vi "Cervena-Narozeninova.vi"(11 "NXT/EV3":T1) -> (3 "NXT/EV3 2":T1)   [LabVIEW 2016]
uses:
  <vilib>/NXT/Subs/LVHSConnector.ctl
  <vilib>/NXT/LegoClasses/BrickReference/BrickReference.lvclass
  <vilib>/NXT/Dual Mode Library/Sound/PlayG.vi
  <vilib>/NXT/Dual Mode Library/Sound/PlayF.vi
  <vilib>/NXT/Dual Mode Library/Sound/PlayE.vi
  <vilib>/NXT/Dual Mode Library/Waits/Wait_Num.vi
  <vilib>/NXT/Dual Mode Library/Sound/PlayA.vi
  <vilib>/NXT/Dual Mode Library/Sound/PlayB.vi
  <vilib>/NXT/Dual Mode Library/Sound/PlayC.vi
  <vilib>/NXT/Dual Mode Library/Sound/PlayD.vi
  <vilib>/NXT/Dual Mode Library/Display/drawText_Center.vi
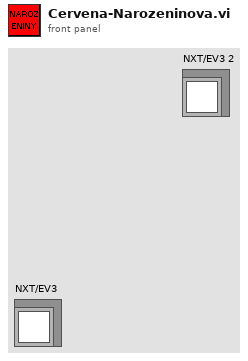
[diagram p1: front panel]
types:
  T1 = typedef "LVHSConnector.ctl" = refnum<class "BrickReference.lvclass">
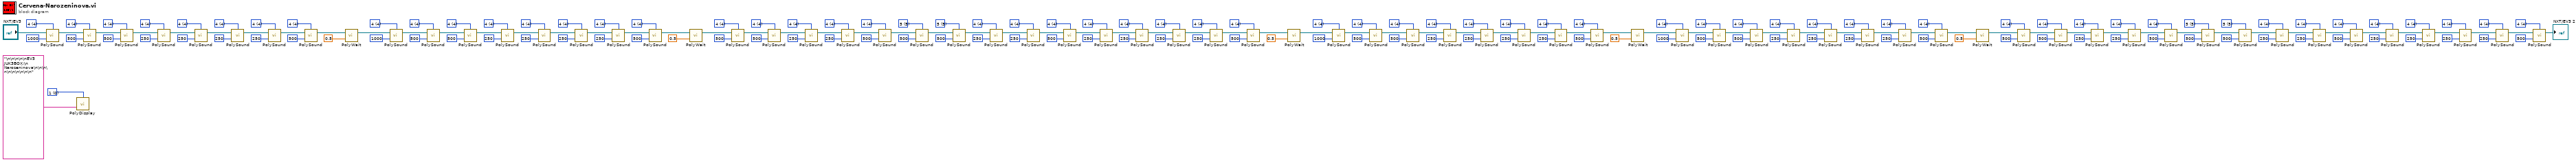
[diagram p0: block diagram]
diagram:
  w1 = i16 0 items=["1", "2", "3", "4", "5", "6", "7", "8", "9", "10", "11", "12"] ("Line")
  w11 = u16 4 items=["3"=3, "4"=4, "5"=5, "6"=6, "7"=7] ("Octave")
  w17 = u16 4 items=["3"=3, "4"=4, "5"=5, "6"=6, "7"=7] ("Octave")
  w16 = u16 4 items=["3"=3, "4"=4, "5"=5, "6"=6, "7"=7] ("Octave")
  w18 = u16 4 items=["3"=3, "4"=4, "5"=5, "6"=6, "7"=7] ("Octave")
  w19 = u16 4 items=["3"=3, "4"=4, "5"=5, "6"=6, "7"=7] ("Octave")
  w27 = u16 4 items=["3"=3, "4"=4, "5"=5, "6"=6, "7"=7] ("Octave")
  w28 = u16 4 items=["3"=3, "4"=4, "5"=5, "6"=6, "7"=7] ("Octave")
  w31 = u16 4 items=["3"=3, "4"=4, "5"=5, "6"=6, "7"=7] ("Octave")
  w33 = u16 5 items=["3"=3, "4"=4, "5"=5, "6"=6, "7"=7] ("Octave")
  w45 = u16 5 items=["3"=3, "4"=4, "5"=5, "6"=6, "7"=7] ("Octave")
  w46 = u16 4 items=["3"=3, "4"=4, "5"=5, "6"=6, "7"=7] ("Octave")
  w49 = u16 4 items=["3"=3, "4"=4, "5"=5, "6"=6, "7"=7] ("Octave")
  w50 = u16 4 items=["3"=3, "4"=4, "5"=5, "6"=6, "7"=7] ("Octave")
  w52 = u16 4 items=["3"=3, "4"=4, "5"=5, "6"=6, "7"=7] ("Octave")
  w55 = u16 4 items=["3"=3, "4"=4, "5"=5, "6"=6, "7"=7] ("Octave")
  w79 = u16 4 items=["3"=3, "4"=4, "5"=5, "6"=6, "7"=7] ("Octave")
  w73 = u16 4 items=["3"=3, "4"=4, "5"=5, "6"=6, "7"=7] ("Octave")
  w72 = u16 4 items=["3"=3, "4"=4, "5"=5, "6"=6, "7"=7] ("Octave")
  w68 = u16 4 items=["3"=3, "4"=4, "5"=5, "6"=6, "7"=7] ("Octave")
  w69 = u16 4 items=["3"=3, "4"=4, "5"=5, "6"=6, "7"=7] ("Octave")
  w62 = u16 4 items=["3"=3, "4"=4, "5"=5, "6"=6, "7"=7] ("Octave")
  w61 = u16 4 items=["3"=3, "4"=4, "5"=5, "6"=6, "7"=7] ("Octave")
  w58 = u16 4 items=["3"=3, "4"=4, "5"=5, "6"=6, "7"=7] ("Octave")
  w82 = u16 4 items=["3"=3, "4"=4, "5"=5, "6"=6, "7"=7] ("Octave")
  w88 = u16 4 items=["3"=3, "4"=4, "5"=5, "6"=6, "7"=7] ("Octave")
  w89 = u16 4 items=["3"=3, "4"=4, "5"=5, "6"=6, "7"=7] ("Octave")
  w93 = u16 4 items=["3"=3, "4"=4, "5"=5, "6"=6, "7"=7] ("Octave")
  w92 = u16 4 items=["3"=3, "4"=4, "5"=5, "6"=6, "7"=7] ("Octave")
  w99 = u16 4 items=["3"=3, "4"=4, "5"=5, "6"=6, "7"=7] ("Octave")
  w100 = u16 4 items=["3"=3, "4"=4, "5"=5, "6"=6, "7"=7] ("Octave")
  w103 = u16 4 items=["3"=3, "4"=4, "5"=5, "6"=6, "7"=7] ("Octave")
  w107 = u16 4 items=["3"=3, "4"=4, "5"=5, "6"=6, "7"=7] ("Octave")
  w113 = u16 4 items=["3"=3, "4"=4, "5"=5, "6"=6, "7"=7] ("Octave")
  w112 = u16 4 items=["3"=3, "4"=4, "5"=5, "6"=6, "7"=7] ("Octave")
  w114 = u16 4 items=["3"=3, "4"=4, "5"=5, "6"=6, "7"=7] ("Octave")
  w115 = u16 4 items=["3"=3, "4"=4, "5"=5, "6"=6, "7"=7] ("Octave")
  w123 = u16 4 items=["3"=3, "4"=4, "5"=5, "6"=6, "7"=7] ("Octave")
  w124 = u16 4 items=["3"=3, "4"=4, "5"=5, "6"=6, "7"=7] ("Octave")
  w127 = u16 4 items=["3"=3, "4"=4, "5"=5, "6"=6, "7"=7] ("Octave")
  w129 = u16 5 items=["3"=3, "4"=4, "5"=5, "6"=6, "7"=7] ("Octave")
  w141 = u16 5 items=["3"=3, "4"=4, "5"=5, "6"=6, "7"=7] ("Octave")
  w142 = u16 4 items=["3"=3, "4"=4, "5"=5, "6"=6, "7"=7] ("Octave")
  w145 = u16 4 items=["3"=3, "4"=4, "5"=5, "6"=6, "7"=7] ("Octave")
  w146 = u16 4 items=["3"=3, "4"=4, "5"=5, "6"=6, "7"=7] ("Octave")
  w148 = u16 4 items=["3"=3, "4"=4, "5"=5, "6"=6, "7"=7] ("Octave")
  w151 = u16 4 items=["3"=3, "4"=4, "5"=5, "6"=6, "7"=7] ("Octave")
  w175 = u16 4 items=["3"=3, "4"=4, "5"=5, "6"=6, "7"=7] ("Octave")
  w169 = u16 4 items=["3"=3, "4"=4, "5"=5, "6"=6, "7"=7] ("Octave")
  w168 = u16 4 items=["3"=3, "4"=4, "5"=5, "6"=6, "7"=7] ("Octave")
  w164 = u16 4 items=["3"=3, "4"=4, "5"=5, "6"=6, "7"=7] ("Octave")
  w165 = u16 4 items=["3"=3, "4"=4, "5"=5, "6"=6, "7"=7] ("Octave")
  w158 = u16 4 items=["3"=3, "4"=4, "5"=5, "6"=6, "7"=7] ("Octave")
  w157 = u16 4 items=["3"=3, "4"=4, "5"=5, "6"=6, "7"=7] ("Octave")
  w154 = u16 4 items=["3"=3, "4"=4, "5"=5, "6"=6, "7"=7] ("Octave")
  w178 = u16 4 items=["3"=3, "4"=4, "5"=5, "6"=6, "7"=7] ("Octave")
  w184 = u16 4 items=["3"=3, "4"=4, "5"=5, "6"=6, "7"=7] ("Octave")
  w185 = u16 4 items=["3"=3, "4"=4, "5"=5, "6"=6, "7"=7] ("Octave")
  w189 = u16 4 items=["3"=3, "4"=4, "5"=5, "6"=6, "7"=7] ("Octave")
  w188 = u16 4 items=["3"=3, "4"=4, "5"=5, "6"=6, "7"=7] ("Octave")
  w195 = u16 4 items=["3"=3, "4"=4, "5"=5, "6"=6, "7"=7] ("Octave")
  w196 = u16 4 items=["3"=3, "4"=4, "5"=5, "6"=6, "7"=7] ("Octave")
  w199 = u16 4 items=["3"=3, "4"=4, "5"=5, "6"=6, "7"=7] ("Octave")
  n1 = call-poly <vilib>:"PolySound.vi"("Duration (500 ms)"=u16 1000, "NXT/EV3"="NXT/EV3", "Octave"=w199) -> ("NXT/EV3"=w193:T1)  [unwired: 1 in]
  n2 = call-poly <vilib>:"PolyDisplay.vi"("Text"="\n\n\n\n\nEV3 JUK3BOX:\n Narozeninova\n\n\n\n\n\n\n\n\n\n", "Line"=w1) -> ()  [unwired: 2 in, 1 out]
  n3 = call-poly <vilib>:"PolySound.vi"("Duration (500 ms)"=u16 500, "NXT/EV3"=w193, "Octave"=w196) -> ("NXT/EV3"=w192:T1)  [unwired: 1 in]
  n4 = call-poly <vilib>:"PolySound.vi"("Duration (500 ms)"=u16 500, "NXT/EV3"=w192, "Octave"=w195) -> ("NXT/EV3"=w180:T1)  [unwired: 1 in]
  n5 = call-poly <vilib>:"PolySound.vi"("Duration (500 ms)"=u16 250, "NXT/EV3"=w180, "Octave"=w188) -> ("NXT/EV3"=w191:T1)  [unwired: 1 in]
  n6 = call-poly <vilib>:"PolySound.vi"("Duration (500 ms)"=u16 250, "NXT/EV3"=w191, "Octave"=w189) -> ("NXT/EV3"=w181:T1)  [unwired: 1 in]
  n7 = call-poly <vilib>:"PolySound.vi"("Duration (500 ms)"=u16 250, "NXT/EV3"=w181, "Octave"=w185) -> ("NXT/EV3"=w182:T1)  [unwired: 1 in]
  n8 = call-poly <vilib>:"PolySound.vi"("Duration (500 ms)"=u16 250, "NXT/EV3"=w182, "Octave"=w184) -> ("NXT/EV3"=w177:T1)  [unwired: 1 in]
  n9 = call-poly <vilib>:"PolySound.vi"("Duration (500 ms)"=u16 500, "NXT/EV3"=w177, "Octave"=w178) -> ("NXT/EV3"=w131:T1)  [unwired: 1 in]
  n10 = call-poly <vilib>:"PolyWait.vi"("Time (1 sec)"=sgl 0.5, "NXT/EV3"=w131) -> ("NXT/EV3"=w153:T1)  [unwired: 2 in]
  n11 = call-poly <vilib>:"PolySound.vi"("Duration (500 ms)"=u16 1000, "NXT/EV3"=w153, "Octave"=w154) -> ("NXT/EV3"=w160:T1)  [unwired: 1 in]
  n12 = call-poly <vilib>:"PolySound.vi"("Duration (500 ms)"=u16 500, "NXT/EV3"=w160, "Octave"=w157) -> ("NXT/EV3"=w161:T1)  [unwired: 1 in]
  n13 = call-poly <vilib>:"PolySound.vi"("Duration (500 ms)"=u16 500, "NXT/EV3"=w161, "Octave"=w158) -> ("NXT/EV3"=w173:T1)  [unwired: 1 in]
  n14 = call-poly <vilib>:"PolySound.vi"("Duration (500 ms)"=u16 250, "NXT/EV3"=w173, "Octave"=w165) -> ("NXT/EV3"=w162:T1)  [unwired: 1 in]
  n15 = call-poly <vilib>:"PolySound.vi"("Duration (500 ms)"=u16 250, "NXT/EV3"=w162, "Octave"=w164) -> ("NXT/EV3"=w172:T1)  [unwired: 1 in]
  n16 = call-poly <vilib>:"PolySound.vi"("Duration (500 ms)"=u16 250, "NXT/EV3"=w172, "Octave"=w168) -> ("NXT/EV3"=w171:T1)  [unwired: 1 in]
  n17 = call-poly <vilib>:"PolySound.vi"("Duration (500 ms)"=u16 250, "NXT/EV3"=w171, "Octave"=w169) -> ("NXT/EV3"=w176:T1)  [unwired: 1 in]
  n18 = call-poly <vilib>:"PolySound.vi"("Duration (500 ms)"=u16 500, "NXT/EV3"=w176, "Octave"=w175) -> ("NXT/EV3"=w133:T1)  [unwired: 1 in]
  n19 = call-poly <vilib>:"PolyWait.vi"("Time (1 sec)"=sgl 0.5, "NXT/EV3"=w133) -> ("NXT/EV3"=w132:T1)  [unwired: 2 in]
  n20 = call-poly <vilib>:"PolySound.vi"("Duration (500 ms)"=u16 500, "NXT/EV3"=w132, "Octave"=w151) -> ("NXT/EV3"=w139:T1)  [unwired: 1 in]
  n21 = call-poly <vilib>:"PolySound.vi"("Duration (500 ms)"=u16 500, "NXT/EV3"=w139, "Octave"=w148) -> ("NXT/EV3"=w138:T1)  [unwired: 1 in]
  n22 = call-poly <vilib>:"PolySound.vi"("Duration (500 ms)"=u16 250, "NXT/EV3"=w138, "Octave"=w146) -> ("NXT/EV3"=w137:T1)  [unwired: 1 in]
  n23 = call-poly <vilib>:"PolySound.vi"("Duration (500 ms)"=u16 250, "NXT/EV3"=w137, "Octave"=w145) -> ("NXT/EV3"=w136:T1)  [unwired: 1 in]
  n24 = call-poly <vilib>:"PolySound.vi"("Duration (500 ms)"=u16 500, "NXT/EV3"=w136, "Octave"=w142) -> ("NXT/EV3"=w135:T1)  [unwired: 1 in]
  n25 = call-poly <vilib>:"PolySound.vi"("Duration (500 ms)"=u16 500, "NXT/EV3"=w135, "Octave"=w141) -> ("NXT/EV3"=w128:T1)  [unwired: 1 in]
  n26 = call-poly <vilib>:"PolySound.vi"("Duration (500 ms)"=u16 500, "NXT/EV3"=w128, "Octave"=w129) -> ("NXT/EV3"=w121:T1)  [unwired: 1 in]
  n27 = call-poly <vilib>:"PolySound.vi"("Duration (500 ms)"=u16 250, "NXT/EV3"=w121, "Octave"=w127) -> ("NXT/EV3"=w120:T1)  [unwired: 1 in]
  n28 = call-poly <vilib>:"PolySound.vi"("Duration (500 ms)"=u16 250, "NXT/EV3"=w120, "Octave"=w124) -> ("NXT/EV3"=w119:T1)  [unwired: 1 in]
  n29 = call-poly <vilib>:"PolySound.vi"("Duration (500 ms)"=u16 500, "NXT/EV3"=w119, "Octave"=w123) -> ("NXT/EV3"=w106:T1)  [unwired: 1 in]
  n30 = call-poly <vilib>:"PolySound.vi"("Duration (500 ms)"=u16 250, "NXT/EV3"=w106, "Octave"=w115) -> ("NXT/EV3"=w118:T1)  [unwired: 1 in]
  n31 = call-poly <vilib>:"PolySound.vi"("Duration (500 ms)"=u16 250, "NXT/EV3"=w118, "Octave"=w114) -> ("NXT/EV3"=w105:T1)  [unwired: 1 in]
  n32 = call-poly <vilib>:"PolySound.vi"("Duration (500 ms)"=u16 250, "NXT/EV3"=w105, "Octave"=w112) -> ("NXT/EV3"=w109:T1)  [unwired: 1 in]
  n33 = call-poly <vilib>:"PolySound.vi"("Duration (500 ms)"=u16 250, "NXT/EV3"=w109, "Octave"=w113) -> ("NXT/EV3"=w104:T1)  [unwired: 1 in]
  n34 = call-poly <vilib>:"PolySound.vi"("Duration (500 ms)"=u16 500, "NXT/EV3"=w104, "Octave"=w107) -> ("NXT/EV3"=w7:T1)  [unwired: 1 in]
  n35 = call-poly <vilib>:"PolyWait.vi"("Time (1 sec)"=sgl 0.5, "NXT/EV3"=w7) -> ("NXT/EV3"=w6:T1)  [unwired: 2 in]
  n36 = call-poly <vilib>:"PolySound.vi"("Duration (500 ms)"=u16 1000, "NXT/EV3"=w6, "Octave"=w103) -> ("NXT/EV3"=w97:T1)  [unwired: 1 in]
  n37 = call-poly <vilib>:"PolySound.vi"("Duration (500 ms)"=u16 500, "NXT/EV3"=w97, "Octave"=w100) -> ("NXT/EV3"=w96:T1)  [unwired: 1 in]
  n38 = call-poly <vilib>:"PolySound.vi"("Duration (500 ms)"=u16 500, "NXT/EV3"=w96, "Octave"=w99) -> ("NXT/EV3"=w84:T1)  [unwired: 1 in]
  n39 = call-poly <vilib>:"PolySound.vi"("Duration (500 ms)"=u16 250, "NXT/EV3"=w84, "Octave"=w92) -> ("NXT/EV3"=w95:T1)  [unwired: 1 in]
  n40 = call-poly <vilib>:"PolySound.vi"("Duration (500 ms)"=u16 250, "NXT/EV3"=w95, "Octave"=w93) -> ("NXT/EV3"=w85:T1)  [unwired: 1 in]
  n41 = call-poly <vilib>:"PolySound.vi"("Duration (500 ms)"=u16 250, "NXT/EV3"=w85, "Octave"=w89) -> ("NXT/EV3"=w86:T1)  [unwired: 1 in]
  n42 = call-poly <vilib>:"PolySound.vi"("Duration (500 ms)"=u16 250, "NXT/EV3"=w86, "Octave"=w88) -> ("NXT/EV3"=w81:T1)  [unwired: 1 in]
  n43 = call-poly <vilib>:"PolySound.vi"("Duration (500 ms)"=u16 500, "NXT/EV3"=w81, "Octave"=w82) -> ("NXT/EV3"=w35:T1)  [unwired: 1 in]
  n44 = call-poly <vilib>:"PolyWait.vi"("Time (1 sec)"=sgl 0.5, "NXT/EV3"=w35) -> ("NXT/EV3"=w57:T1)  [unwired: 2 in]
  n45 = call-poly <vilib>:"PolySound.vi"("Duration (500 ms)"=u16 1000, "NXT/EV3"=w57, "Octave"=w58) -> ("NXT/EV3"=w64:T1)  [unwired: 1 in]
  n46 = call-poly <vilib>:"PolySound.vi"("Duration (500 ms)"=u16 500, "NXT/EV3"=w64, "Octave"=w61) -> ("NXT/EV3"=w65:T1)  [unwired: 1 in]
  n47 = call-poly <vilib>:"PolySound.vi"("Duration (500 ms)"=u16 500, "NXT/EV3"=w65, "Octave"=w62) -> ("NXT/EV3"=w77:T1)  [unwired: 1 in]
  n48 = call-poly <vilib>:"PolySound.vi"("Duration (500 ms)"=u16 250, "NXT/EV3"=w77, "Octave"=w69) -> ("NXT/EV3"=w66:T1)  [unwired: 1 in]
  n49 = call-poly <vilib>:"PolySound.vi"("Duration (500 ms)"=u16 250, "NXT/EV3"=w66, "Octave"=w68) -> ("NXT/EV3"=w76:T1)  [unwired: 1 in]
  n50 = call-poly <vilib>:"PolySound.vi"("Duration (500 ms)"=u16 250, "NXT/EV3"=w76, "Octave"=w72) -> ("NXT/EV3"=w75:T1)  [unwired: 1 in]
  n51 = call-poly <vilib>:"PolySound.vi"("Duration (500 ms)"=u16 250, "NXT/EV3"=w75, "Octave"=w73) -> ("NXT/EV3"=w80:T1)  [unwired: 1 in]
  n52 = call-poly <vilib>:"PolySound.vi"("Duration (500 ms)"=u16 500, "NXT/EV3"=w80, "Octave"=w79) -> ("NXT/EV3"=w37:T1)  [unwired: 1 in]
  n53 = call-poly <vilib>:"PolyWait.vi"("Time (1 sec)"=sgl 0.5, "NXT/EV3"=w37) -> ("NXT/EV3"=w36:T1)  [unwired: 2 in]
  n54 = call-poly <vilib>:"PolySound.vi"("Duration (500 ms)"=u16 500, "NXT/EV3"=w36, "Octave"=w55) -> ("NXT/EV3"=w43:T1)  [unwired: 1 in]
  n55 = call-poly <vilib>:"PolySound.vi"("Duration (500 ms)"=u16 500, "NXT/EV3"=w43, "Octave"=w52) -> ("NXT/EV3"=w42:T1)  [unwired: 1 in]
  n56 = call-poly <vilib>:"PolySound.vi"("Duration (500 ms)"=u16 250, "NXT/EV3"=w42, "Octave"=w50) -> ("NXT/EV3"=w41:T1)  [unwired: 1 in]
  n57 = call-poly <vilib>:"PolySound.vi"("Duration (500 ms)"=u16 250, "NXT/EV3"=w41, "Octave"=w49) -> ("NXT/EV3"=w40:T1)  [unwired: 1 in]
  n58 = call-poly <vilib>:"PolySound.vi"("Duration (500 ms)"=u16 500, "NXT/EV3"=w40, "Octave"=w46) -> ("NXT/EV3"=w39:T1)  [unwired: 1 in]
  n59 = call-poly <vilib>:"PolySound.vi"("Duration (500 ms)"=u16 500, "NXT/EV3"=w39, "Octave"=w45) -> ("NXT/EV3"=w32:T1)  [unwired: 1 in]
  n60 = call-poly <vilib>:"PolySound.vi"("Duration (500 ms)"=u16 500, "NXT/EV3"=w32, "Octave"=w33) -> ("NXT/EV3"=w25:T1)  [unwired: 1 in]
  n61 = call-poly <vilib>:"PolySound.vi"("Duration (500 ms)"=u16 250, "NXT/EV3"=w25, "Octave"=w31) -> ("NXT/EV3"=w24:T1)  [unwired: 1 in]
  n62 = call-poly <vilib>:"PolySound.vi"("Duration (500 ms)"=u16 250, "NXT/EV3"=w24, "Octave"=w28) -> ("NXT/EV3"=w23:T1)  [unwired: 1 in]
  n63 = call-poly <vilib>:"PolySound.vi"("Duration (500 ms)"=u16 500, "NXT/EV3"=w23, "Octave"=w27) -> ("NXT/EV3"=w10:T1)  [unwired: 1 in]
  n64 = call-poly <vilib>:"PolySound.vi"("Duration (500 ms)"=u16 250, "NXT/EV3"=w10, "Octave"=w19) -> ("NXT/EV3"=w22:T1)  [unwired: 1 in]
  n65 = call-poly <vilib>:"PolySound.vi"("Duration (500 ms)"=u16 250, "NXT/EV3"=w22, "Octave"=w18) -> ("NXT/EV3"=w9:T1)  [unwired: 1 in]
  n66 = call-poly <vilib>:"PolySound.vi"("Duration (500 ms)"=u16 250, "NXT/EV3"=w9, "Octave"=w16) -> ("NXT/EV3"=w13:T1)  [unwired: 1 in]
  n67 = call-poly <vilib>:"PolySound.vi"("Duration (500 ms)"=u16 250, "NXT/EV3"=w13, "Octave"=w17) -> ("NXT/EV3"=w8:T1)  [unwired: 1 in]
  n68 = call-poly <vilib>:"PolySound.vi"("Duration (500 ms)"=u16 500, "NXT/EV3"=w8, "Octave"=w11) -> ("NXT/EV3"=→"NXT/EV3 2":T1)  [unwired: 1 in]
